vi "02_DATA_loop.vi"(9 "Data queue":refnum<queue>, 11 "VISA resource name":refnum<visa-resource-name>) -> ()   [LabVIEW 2017]
panel:
  in  "R_array, Ohm":dbl[](array[numeric])=[5000000000.0, 50000000.0, 510000.0, 5200.0, 400.0, 0.0]
  in  "C_array, F":dbl[](array[numeric])=[0.0, 1e-11, 1e-10, 1e-09, 1e-07, 1e-05]
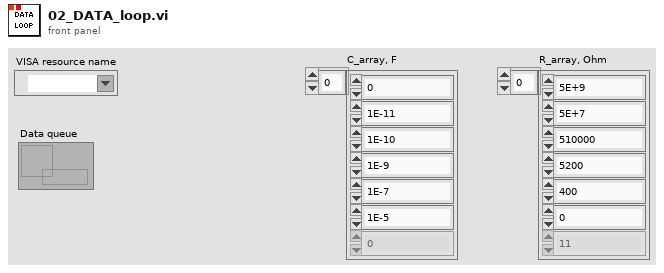
[diagram p1: front panel]
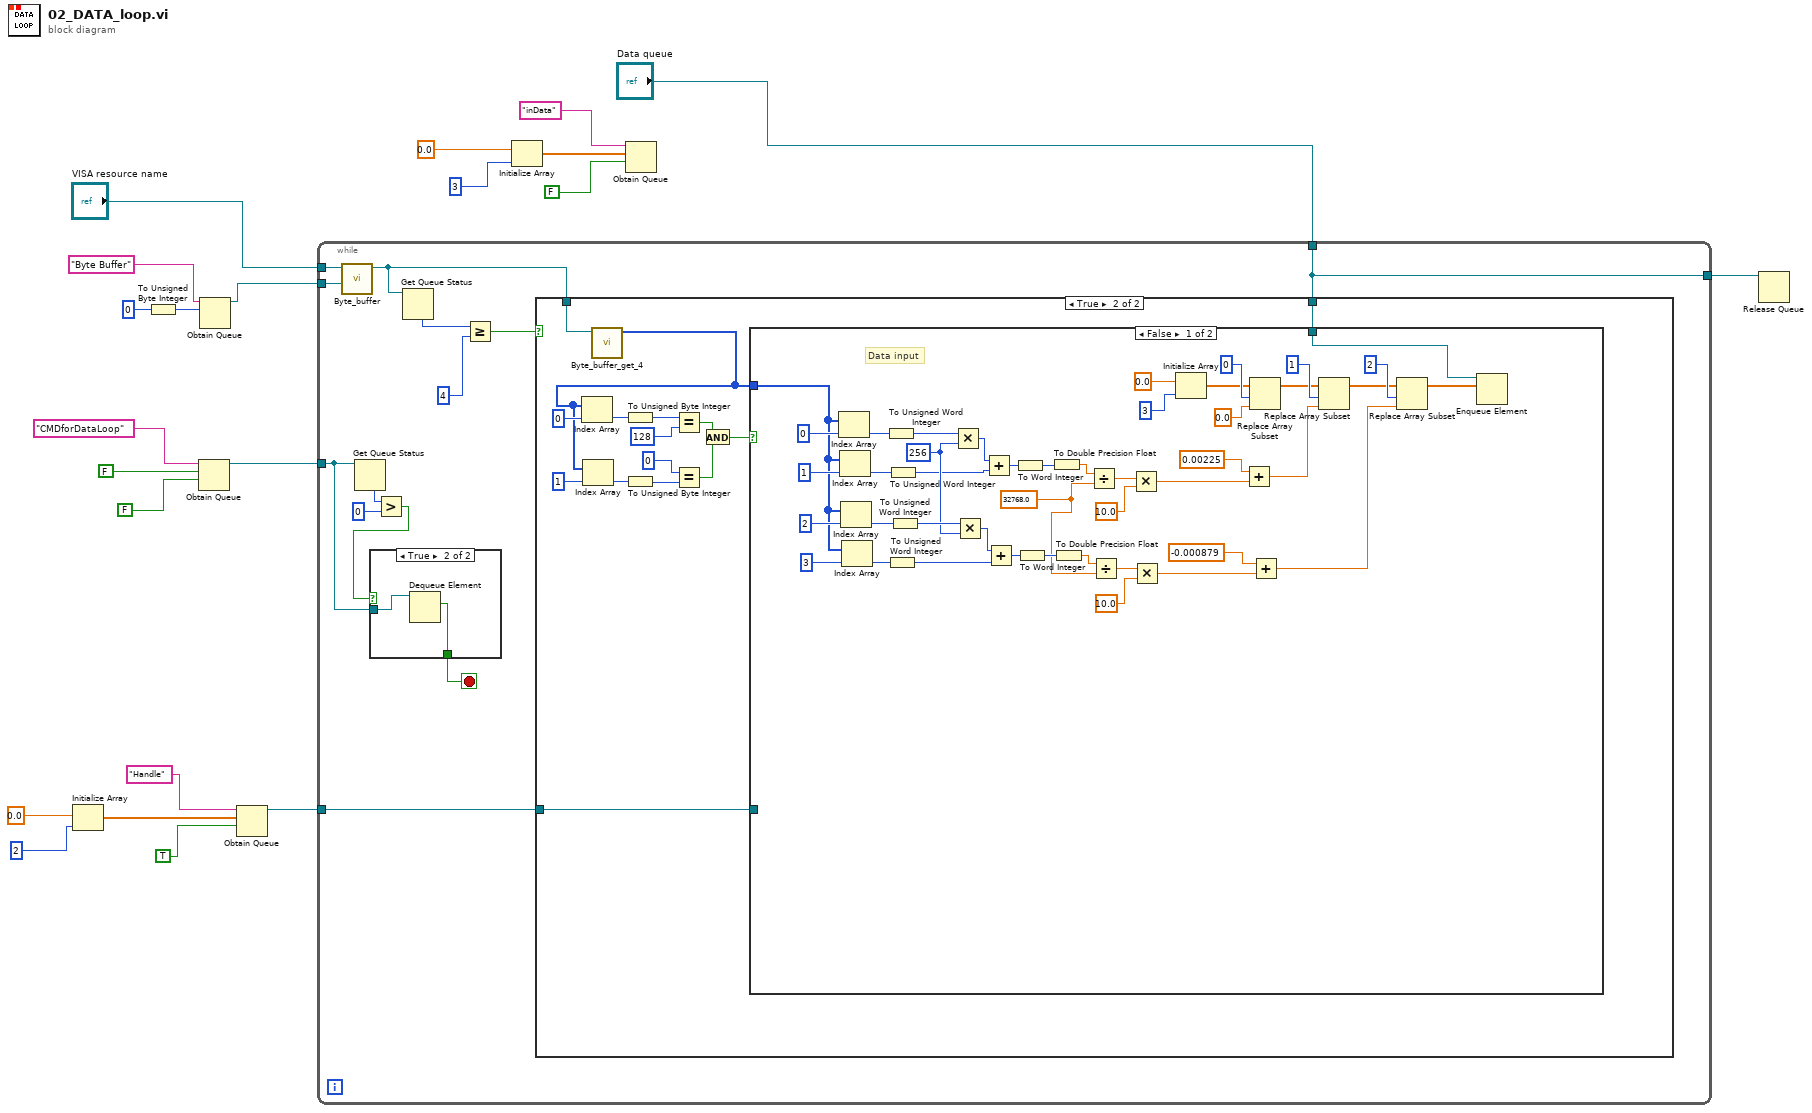
[diagram p0: block diagram]
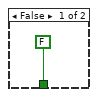
[diagram p2: hidden frame]
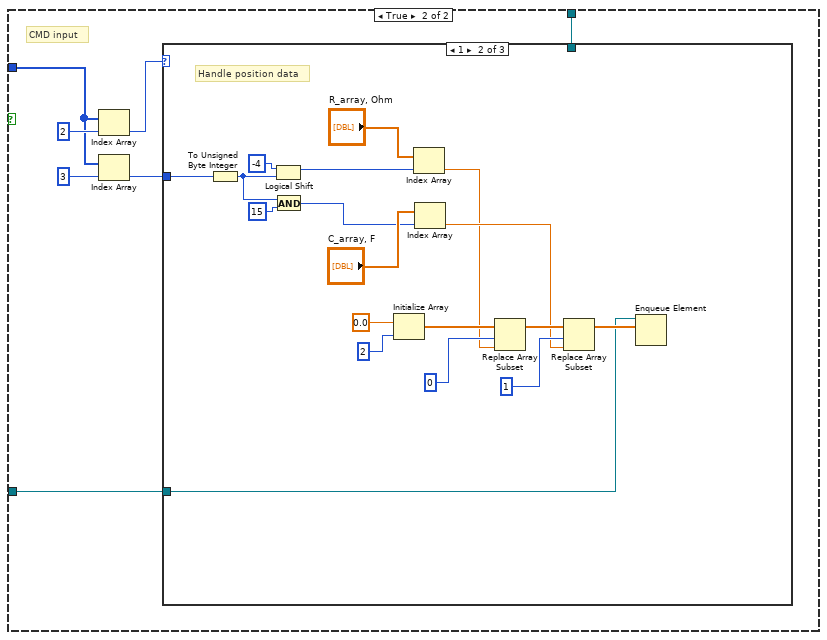
[diagram p4: hidden frame]
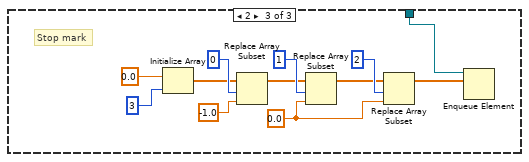
[diagram p6: hidden frame]
diagram:
  n1 = Initialize Array(0.0, 2 ("dimension size")) -> (w10:dbl[])
  n2 = To Unsigned Byte Integer(number=u8 0) -> (unsigned 8bit integer=w4:u8)
  n3 = Obtain Queue(name (unnamed)="CMDforDataLoop", element data type=FALSE ("create if not found? (T)"), create if not found? (T)=FALSE) -> (queue out=w12:refnum<queue>)  [unwired: 2 in, 2 out]
  n4 = Obtain Queue(name (unnamed)="Byte Buffer", element data type=w4) -> (queue out=w1:refnum<queue>)  [unwired: 3 in, 2 out]
  n5 = Obtain Queue(name (unnamed)="Handle", element data type=w10, create if not found? (T)=TRUE) -> (queue out=w5:refnum<queue>)  [unwired: 2 in, 2 out]
  n6 = while {
    tunnel: "VISA resource name" -> [w28]
    tunnel: "Data queue" -> [w34]
    tunnel: [w34] -> w13
    tunnel: w12 -> [w30]
    tunnel: w5 -> [w25]
    tunnel: w1 -> [w24]
    stop <- w29 stop-if-true
    n7 = call "Byte_buffer.vi"("byte queue"=w24, "reference"=w28) -> ("byte queue out"=w23:refnum<queue>)  [unwired: 8 in, 1 out]
    n8 = Get Queue Status(queue=w30) -> (# elements in queue=w33:i32)  [unwired: 2 in, 7 out]
    n9 = Greater?(x=w33, y=0) -> (0:w31:bool)
    n10 = case shown="True" w31 {
      tunnel: w30 -> [_ w38]
      tunnel: [FALSE ("create if not found? (T)") w37] -> w29
      frame False {
      }
      frame True {
        n11 = Dequeue Element(queue=w38) -> (element=w37:bool)  [unwired: 2 in, 3 out]
      }
    }
    n12 = Get Queue Status(queue=w23) -> (# elements in queue=w27:i32)  [unwired: 2 in, 7 out]
    n13 = Greater Or Equal?(x=w27, y=4) -> (x >= y?=w35:bool)
    n14 = case shown="True" w35 {
      tunnel: w34 -> [_ w43]
      tunnel: w23 -> [_ w41]
      tunnel: w25 -> [_ w40]
      frame False {
      }
      frame True {
        n15 = call "Byte_buffer_get_4.vi"("queue out"=w41) -> ("Array"=w42:u8[])  [unwired: 10 in]
        n16 = Index Array(array=w42, index=0) -> (element=w51:u8)
        n17 = Index Array(array=w42, index=1) -> (element=w50:u8)
        n18 = To Unsigned Byte Integer(number=w51) -> (unsigned 8bit integer=w49:u8)
        n19 = To Unsigned Byte Integer(number=w50) -> (unsigned 8bit integer=w48:u8)
        n20 = Equal?(x=w49, y=u8 128) -> (x = y?=w46:bool)
        n21 = Equal?(x=u8 0 ("y"), y=w48) -> (x = y?=w45:bool)
        n22 = And(x=w46, y=w45) -> (x .and. y?=w44:bool)
        n23 = case shown="False" w44 {
          tunnel: w42 -> [w83 w103]
          tunnel: w43 -> [w72 w100]
          tunnel: w40 -> [_ w99]
          frame False {
            w64 = 32768.0 ("y")
            w65 = u16 256 ("y")
            # "Data input"
            n24 = Index Array(array=w83, index=0) -> (element=w71:u8)
            n25 = Index Array(array=w83, index=1) -> (element=w70:u8)
            n26 = Index Array(array=w83, index=2) -> (element=w68:u8)
            n27 = Index Array(array=w83, index=3) -> (element=w69:u8)
            n28 = To Unsigned Word Integer(number=w71) -> (unsigned 16bit integer=w61:u16)
            n29 = To Unsigned Word Integer(number=w69) -> (unsigned 16bit integer=w67:u16)
            n30 = To Unsigned Word Integer(number=w70) -> (unsigned 16bit integer=w60:u16)
            n31 = To Unsigned Word Integer(number=w68) -> (unsigned 16bit integer=w66:u16)
            n32 = Multiply(x=w61, y=w65) -> (x*y=w90:u16)
            n33 = Multiply(x=w66, y=w65) -> (x*y=w91:u16)
            n34 = Add(x=w90, y=w60) -> (x+y=w63:u16)
            n35 = Add(x=w91, y=w67) -> (x+y=w92:u16)
            n36 = To Word Integer(number=w63) -> (16bit integer=w62:i16)
            n37 = To Word Integer(number=w92) -> (16bit integer=w94:i16)
            n38 = To Double Precision Float(number=w62) -> (double precision float=w95:dbl)
            n39 = To Double Precision Float(number=w94) -> (double precision float=w93:dbl)
            n40 = Divide(x=w95, y=w64) -> (x/y=w96:dbl)
            n41 = Divide(x=w93, y=w64) -> (x/y=w97:dbl)
            n42 = Multiply(x=w96, y=10.0) -> (x*y=w58:dbl)
            n43 = Multiply(x=w97, y=10.0) -> (x*y=w57:dbl)
            n44 = Initialize Array(0.0 ("y"), 3 ("dimension size")) -> (w78:dbl[])
            n45 = Add(x=0.00225, y=w58) -> (x+y=w59:dbl)
            n46 = Replace Array Subset(array=w78, new element=0.0 ("new element/subarray"), index=0) -> (w77:dbl[])
            n47 = Add(x=-0.000879, y=w57) -> (x+y=w56:dbl)
            n48 = Replace Array Subset(array=w77, new element=w59, index=1) -> (w75:dbl[])
            n49 = Replace Array Subset(array=w75, new element=w56, index=2) -> (w74:dbl[])
            n50 = Enqueue Element(queue=w72, element=w74) -> ()  [unwired: 2 in, 3 out]
          }
          frame True {
            # "CMD input"
            n51 = Index Array(array=w103, index=2) -> (element=w101:u8)
            n52 = Index Array(array=w103, index=3) -> (element=w98:u8)
            n53 = case shown="1" w101 {
              tunnel: w98 -> [_ w120 _]
              tunnel: w100 -> [_ _ w124]
              tunnel: w99 -> [_ w108 _]
              frame 0, Default {
              }
              frame 1 {
                # "Handle position data"
                n54 = To Unsigned Byte Integer(number=w120) -> (unsigned 8bit integer=w107:u8)
                n55 = Logical Shift(y=i8 -4 ("x"), x=w107) -> (x << y=w117:u8)
                n56 = And(x=w107, y=u8 15) -> (x .and. y?=w116:u8)
                n57 = Initialize Array(0.0 ("y"), 2 ("dimension size")) -> (w110:dbl[])
                n58 = Index Array(array="R_array, Ohm", index=w117) -> (element=w105:dbl)
                n59 = Index Array(array="C_array, F", index=w116) -> (element=w106:dbl)
                n60 = Replace Array Subset(array=w110, new element=w105, index=0) -> (w111:dbl[])
                n61 = Replace Array Subset(array=w111, new element=w106, index=1) -> (w109:dbl[])
                n62 = Enqueue Element(queue=w108, element=w109) -> ()  [unwired: 2 in, 3 out]
              }
              frame 2 {
                w123 = 0.0 ("new element/subarray")
                # "Stop mark"
                n63 = Initialize Array(0.0 ("y"), 3 ("dimension size")) -> (w130:dbl[])
                n64 = Replace Array Subset(array=w130, new element=-1.0 ("new element/subarray"), index=0) -> (w129:dbl[])
                n65 = Replace Array Subset(array=w129, new element=w123, index=1) -> (w127:dbl[])
                n66 = Replace Array Subset(array=w127, new element=w123, index=2) -> (w126:dbl[])
                n67 = Enqueue Element(queue=w124, element=w126) -> ()  [unwired: 2 in, 3 out]
              }
            }
          }
        }
      }
    }
  }
  n68 = Initialize Array(0.0, 3 ("dimension size")) -> (w20:dbl[])
  n69 = Obtain Queue(name (unnamed)="inData", element data type=w20, create if not found? (T)=FALSE) -> ()  [unwired: 2 in, 3 out]
  n70 = Release Queue(queue=w13) -> ()  [unwired: 2 in, 3 out]
